vi "HAL Camera specifications globals.vi"() -> ()   [LabVIEW 2011]
panel:
  in  "Camera Name":string="Andor iXon 512"
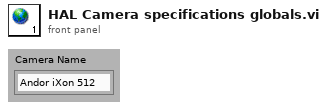
[diagram p1: front panel]
diagram:
